vi "stoperaseXY_img.vi"   [LabVIEW 2013]
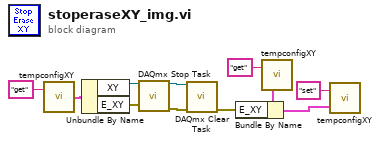
[diagram p0: block diagram]
diagram:
  n1 = call "tempconfigXY.vi"("command"="get") -> ("Temp Config out"=w4:cluster{" XY":refnum<k21>, "E_XY":errorcluster})  [unwired: 1 in]
  n2 = Unbundle By Name(w4) -> ("XY"=w5:refnum<k21>, "E_XY"=w6:errorcluster)
  n3 = call <vilib>:"DAQmx Stop Task.vi"("task/channels in"=w5, "error in"=w6) -> ("task out"=w2:refnum<k21>, "error out"=w1:errorcluster)  [unwired: 12 in]
  n4 = call <vilib>:"DAQmx Clear Task.vi"("task in"=w2, "error in"=w1) -> ("error out"=w10:errorcluster)  [unwired: 13 in]
  n5 = call "tempconfigXY.vi"("command"="get") -> ("Temp Config out"=w9:cluster{" XY":refnum<k21>, "E_XY":errorcluster})  [unwired: 1 in]
  n6 = Bundle By Name(cluster=w9, "E_XY"=w10) -> (w11:cluster{" XY":refnum<k21>, "E_XY":errorcluster})
  n7 = call "tempconfigXY.vi"("Temp Config in"=w11, "command"="set") -> ()  [unwired: 1 out]
